vi "FTW-Tag-SetVariant.vi"(0 "FTW Actor Connector In":refnum<class "FTW-ActorConnector.lvclass">, 5 "Tag Object":variant, 11 "error in (no error)":errorcluster) -> (4 "FTW Actor Connector":refnum<class "FTW-ActorConnector.lvclass">, 14 "Roundtrip Time":dbl format="%.6f sec", 15 "error out":errorcluster)   [LabVIEW 2018]
uses:
  Connector/FTW-ActorConnector.lvclass
  a81fc6b2-6e43-4286-8517-d3fcdad9e5f4.vi
  a81fc6b2-6e43-4286-8517-d3fcdad9e5f4.vi/5315b429-07cc-44c8-bb9b-54570a5dc9d4.vi
  container/FTW-Container-FromVariant.vi
  container/FTW-Container-New-FromContainer.vi
  JSON/FTW-JSON-SerializeAndDestroy.vi
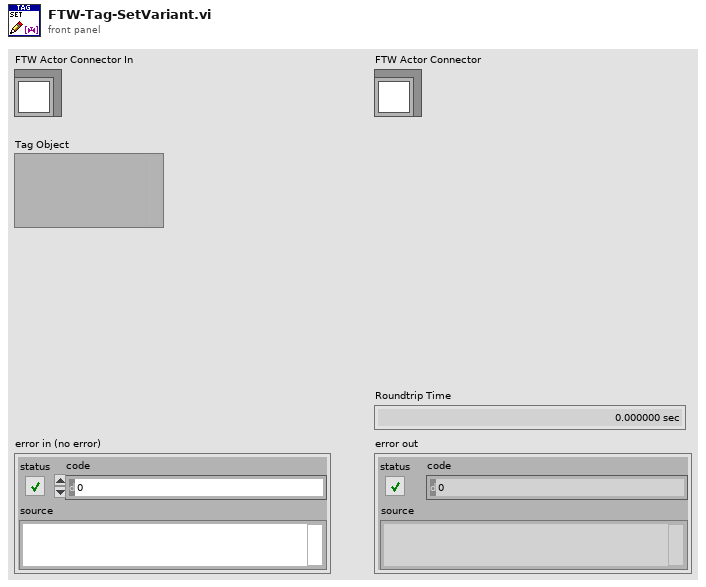
[diagram p1: front panel]
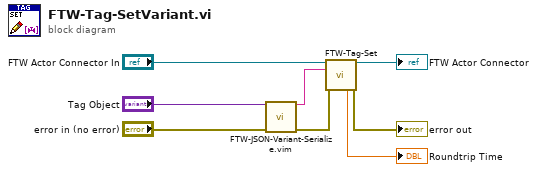
[diagram p0: block diagram]
diagram:
  n1 = call "FTW-JSON-Variant-Serialize.vim"("Variant"="Tag Object", "error in"="error in (no error)") -> ("JSON String"=w2:string, "error out"=w3:errorcluster)  [unwired: 12 in]
  n2 = call "FTW-Tag-Set.vi"("FTW Actor Connector In"="FTW Actor Connector In", "Tag Object"=w2, "error in (no error)"=w3) -> ("FTW Actor Connector"=→"FTW Actor Connector":refnum<class "FTW-ActorConnector.lvclass">, "Roundtrip Time"=→"Roundtrip Time":dbl, "error out"=→"error out":errorcluster)  [unwired: 10 in]
